vi "Calibrate Stereo Vision System (mod).vi"() -> ()   [LabVIEW 2014]
doc: "This example acquires images and demonstrates the binocular stereo vision algorithms installed with NI Vision Development Module. This example requires NI-IMAQdx. Refer to the Detailed Help for more information."
uses:
  SubVIs/Stereo - Calibration Manager Function.ctl
  <vilib>/vision/Stereo.llb/IMAQ Binocular Reference Coordinate System.ctl
  SubVIs/Stereo - Global Variables.vi
  <vilib>/vision/NI_Vision_Development_Module.lvlib
panel:
  in  "Process Band":bool
  out "Unit":string
  in  "Units":string[](array[string])=["", "Angström", "Micrometer", "Millimeter", "Centimeter", "Meter", "Kilometer", "Microinch", "Inch", "Feet", "Nautical miles", "Standard miles", "Steps"]
  out "Depth":dbl caption="Depth:"
  in  "Interpolate Disparity":bool=TRUE
  in  "Overlay Horizontal Lines":bool
  in  "View":enum16{"Acquired Images", "Rectified Images"}(ring)
  out "Grid Descriptor":cluster{"X Step":sgl, "Y Step":sgl, "Unit":T1}={"X Step"=1.0, "Y Step"=1.0, "Unit"=enum."Inch"}
  out "Grid Size":cluster{"X":i32, "Y":i32}
  in  "Live Image":bool=TRUE
  out "Calibration Status":u16(ring)
  in  "Display":enum16{"Disparity Image", "Depth Image"}(ring)
  in  "Relative Coordinate System":T2
  out "Image":sgl[][](graph) caption="Grid Coverage"
  in  "Exit":bool
  in  "Tab Control":T3(tab)
  out "Grid Coverage":T5
  in  "Save Single Calibrations":bool
  out "Quality":T6 caption="Stereo Calibration Quality" {"Rectification Quality 2" format="%#.5g"; "Rectification Quality" format="%#.5g"; "Calibration Quality" format="%#.5g"; "Max Distance" format="%#.4g"}
  in  "Save Grid Images":bool
  out "Scrollbar":u8(slide) caption="Acquire image in..." max=50 scale=0.0..100.0
  in  "Save Stereo Calibration":bool
  in  "Scaling Factor":sgl=1.0 min=0 max=1 step=0.1
  in  "Load":bool
  in  "Calibrate":bool
  out "Instruction Images":u16(ring) caption="Grid Orientation"
  out "Instructions":string
  in  "Time Lapse":u16=4 caption="Image Acquisition Time Lapse" min=1 max=60 step=1
  out "Grid Valid":bool=TRUE
  out "Calibration Grids":cluster{"Left Image":T4, "Right Image":T4}[](array[cluster]) caption="Left Calibration Grids"
  in  "Show":enum16{"Grid Coverage", "Calibration Grids"}(ring)
  in  "Max Depth (SGBM)":sgl=45.0 caption="Maximum Depth"
  in  "Correspondence Options SGBM":T7={"Method"=0, "Window Size"=15.0, "Minimum Disparity"=0.0, "Number of Disparity"=144.0, "P1"=100.0, "P2"=500.0, "Full DP"=FALSE, "Max Left Right Disparity"=5.0, "Subpixel"=TRUE, "Invalid Disparity Replace Value"=-16.0} caption="Correspondence Options" {"Method" items=["SAD"]; "Number of Disparity" min=16.0 step=16.0; "Window Size" min=5.0 max=255.0 step=2.0}
  in  "Postfilter Options SGBM":T8={"Texture Threshold"=0.0, "Uniqueness Ratio"=0.0, "Speckle Window Size"=5.0, "Speckle Range"=200.0} caption="Postfilter Options" {"Speckle Range" min=0.0; "Speckle Window Size" min=0.0; "Uniqueness Ratio" min=0.0 max=100.0; "Texture Threshold" min=0.0}
  in  "Filter Cap":u32=32
  in  "Correspondence Options BM":T9={"Method"=0, "Window Size"=25.0, "Minimum Disparity"=0.0, "Number of Disparity"=144.0, "Left - Right Check"=5.0, "Subpixel"=TRUE, "Invalid Disparity Replace Value"=-16.0} caption="Correspondence Options" {"Method" items=["SAD"]; "Number of Disparity" min=16.0 step=16.0; "Window Size" min=5.0 max=255.0 step=2.0}
  in  "Postfilter Options BM":T8={"Texture Threshold"=0.0, "Uniqueness Ratio"=0.0, "Speckle Window Size"=5.0, "Speckle Range"=200.0} caption="Postfilter Options" {"Speckle Range" min=0.0; "Speckle Window Size" min=0.0; "Uniqueness Ratio" min=0.0 max=100.0 step=1.0; "Texture Threshold" min=0.0}
  in  "Prefilter Options":T10={"Filter Type"=2, "Filter Size"=9.0, "Filter Cap"=31.0} {"Filter Type" items=["None", "Normal Response", "Sobel"]; "Filter Cap" min=1.0 max=63.0 step=1.0; "Filter Size" min=5.0 max=255.0 step=2.0}
  in  "Max Depth (BM)":sgl=45.0 caption="Maximum Depth"
  out "Right Image":T4(plugin-control)
  out "Left Image":T4(plugin-control)
  # "Overview: Demonstrate how to calibrate a stereo system and compute a depth image.\nRequirements: LabVIEW Full Development System, NI-IMAQdx and Vision Development Module\nNote: This example does not run on LabVIEW Real Time"
  # "s"
  # "Right Calibration Grids"
  # "Set the Maximum Depth corresponding to your setting:"
  # "Set the Maximum Depth corresponding to your setting:"
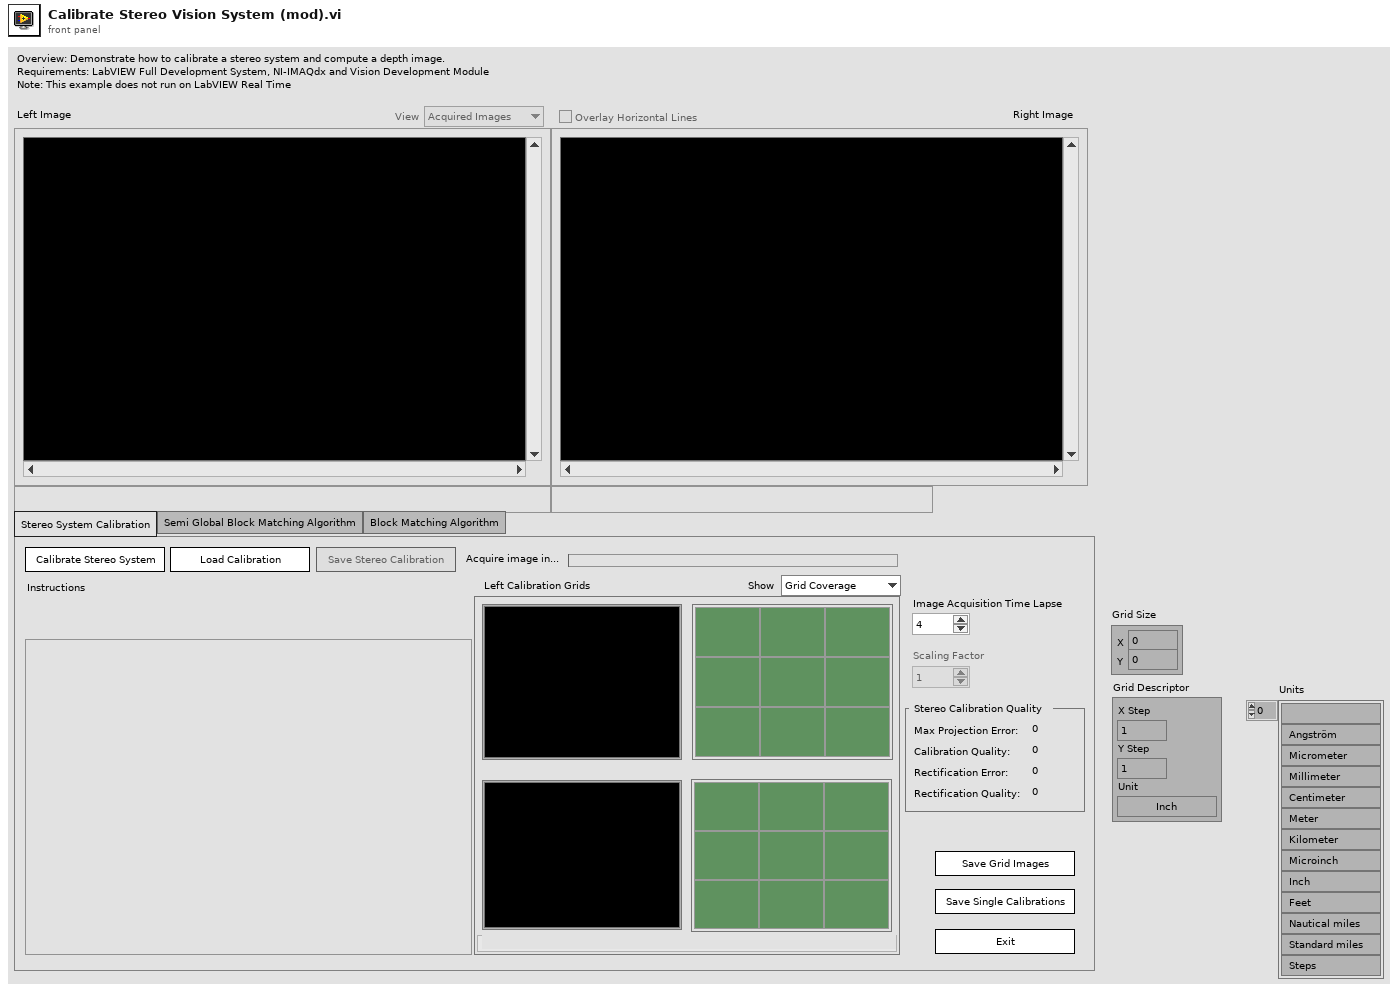
[diagram p1: front panel]
types:
  T1 = typedef "Image Unit" = enum32{"Undefined", "Angström", "Micrometer", "Millimeter", "Centimeter", "Meter", "Kilometer", "Microinch", "Inch", "Feet", "Nautical miles", "Standard miles", "Steps"}
  T2 = cluster{"Translation":cluster{"X":dbl, "Y":dbl, "Z":dbl}, "Rotation":cluster{"X":dbl, "Y":dbl, "Z":dbl}}
  T3 = enum32{"Stereo System Calibration", "Semi Global Block Matching Algorithm", "Block Matching Algorithm"}
  T4 = typedef "IMAQ Image.ctl" = refnum<image>
  T5 = cluster{"Left Image":T4, "Left Grid Coverage":bool[][], "Left Grid Coverage 3":string[][], "Right Image":T4, "Left Grid Coverage 2":bool[][], "Left Grid Coverage 4":string[][]}
  T6 = cluster{"Max Distance":dbl, "Calibration Quality":dbl, "Rectification Quality":dbl, "Rectification Quality 2":dbl}
  T7 = cluster{"Method":u16, "Window Size":dbl, "Minimum Disparity":dbl, "Number of Disparity":dbl, "P1":dbl, "P2":dbl, "Full DP":bool, "Max Left Right Disparity":dbl, "Subpixel":bool, "Invalid Disparity Replace Value":dbl}
  T8 = cluster{"Texture Threshold":dbl, "Uniqueness Ratio":dbl, "Speckle Window Size":dbl, "Speckle Range":dbl}
  T9 = cluster{"Method":u16, "Window Size":dbl, "Minimum Disparity":dbl, "Number of Disparity":dbl, "Left - Right Check":dbl, "Subpixel":bool, "Invalid Disparity Replace Value":dbl}
  T10 = cluster{"Filter Type":u16, "Filter Size":dbl, "Filter Cap":dbl}
  T11 = typedef "Stereo - Calibration Manager Function.ctl" = enum16{"Init", "Add Grid Images", "Get Images", "Dispose"}
  T12 = enum32{"Zero Order", "Bilinear", "Quadratic", "Cubic", "Bilinear Fixed"}
  T13 = typedef "IMAQ Binocular Reference Coordinate System.ctl" = enum32{" Left Camera", "Right Camera"}
  T14 = cluster{"Learn Lookup Table?":bool, "Render to original image?":bool, "Scaling Factor":sgl}
  T15 = enum8{"Enabled", "Disabled", "Disabled and Grayed Out"}
  T16 = enum32{"Page Enabled", "Page Disabled", "Page Disabled & Grayed"}
  T17 = typedef "Image Type" = u32
  T18 = typedef "IMAQ Binocular Stereo Session.ctl" = refnum<k1>
  T19 = typedef "Calibration Reference Points.ctl" = cluster{"Pixel Coordinates":cluster{"X":dbl, "Y":dbl}[], "Real World Coordinates":cluster{"X":dbl, "Y":dbl}[], "Unit":T1, "Image Size":cluster{"X":u32, "Y":u32}}
  T20 = cluster{"Image (dup)":T4, "Reference Points":T19}
  T21 = cluster{"Max. Projection Error":dbl, "Calibration Quality":dbl, "Max. Rectification Error":dbl, "Rectification Quality":dbl}
  T22 = typedef "LVPoint32TypeDef.ctl" = cluster{"Horizontal":i32, "Vertical":i32}
  T23 = cluster{"Max Depth (BM)":sgl, "Max Depth (BM)":sgl}
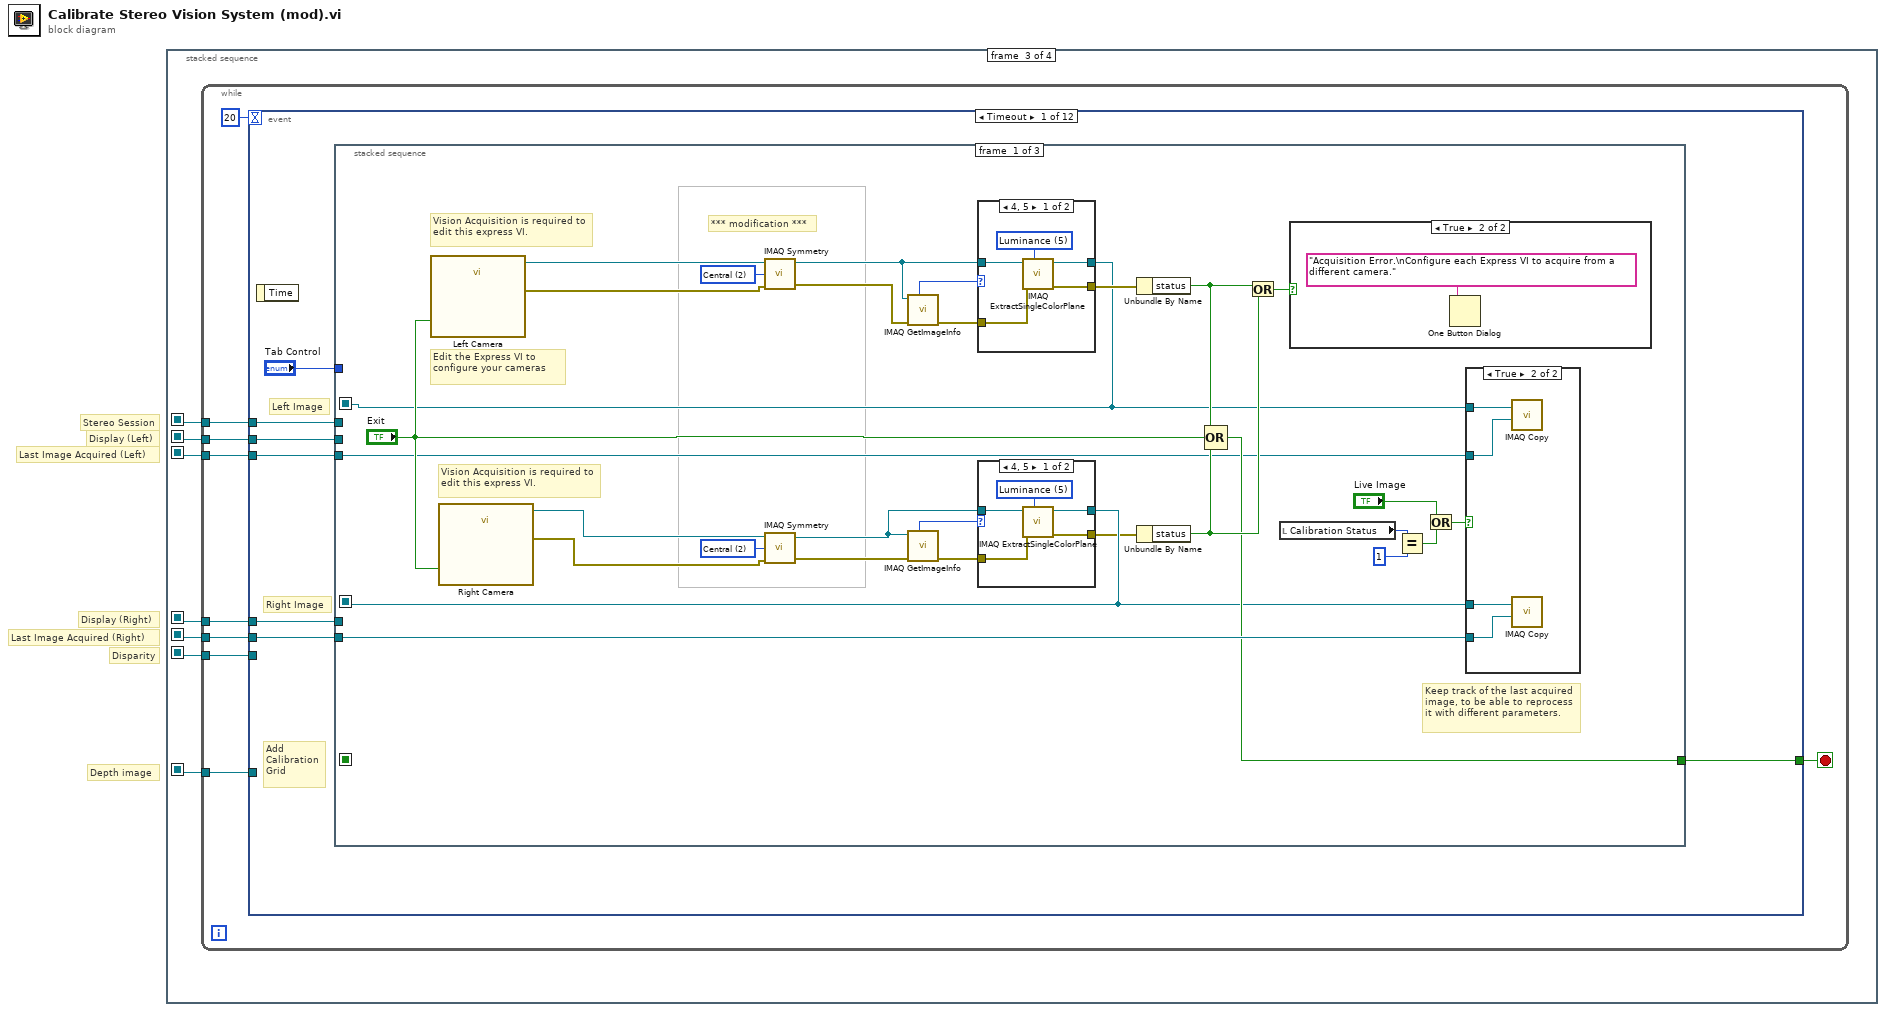
[diagram p0: block diagram]
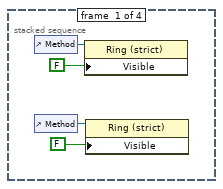
[diagram p2: hidden frame]
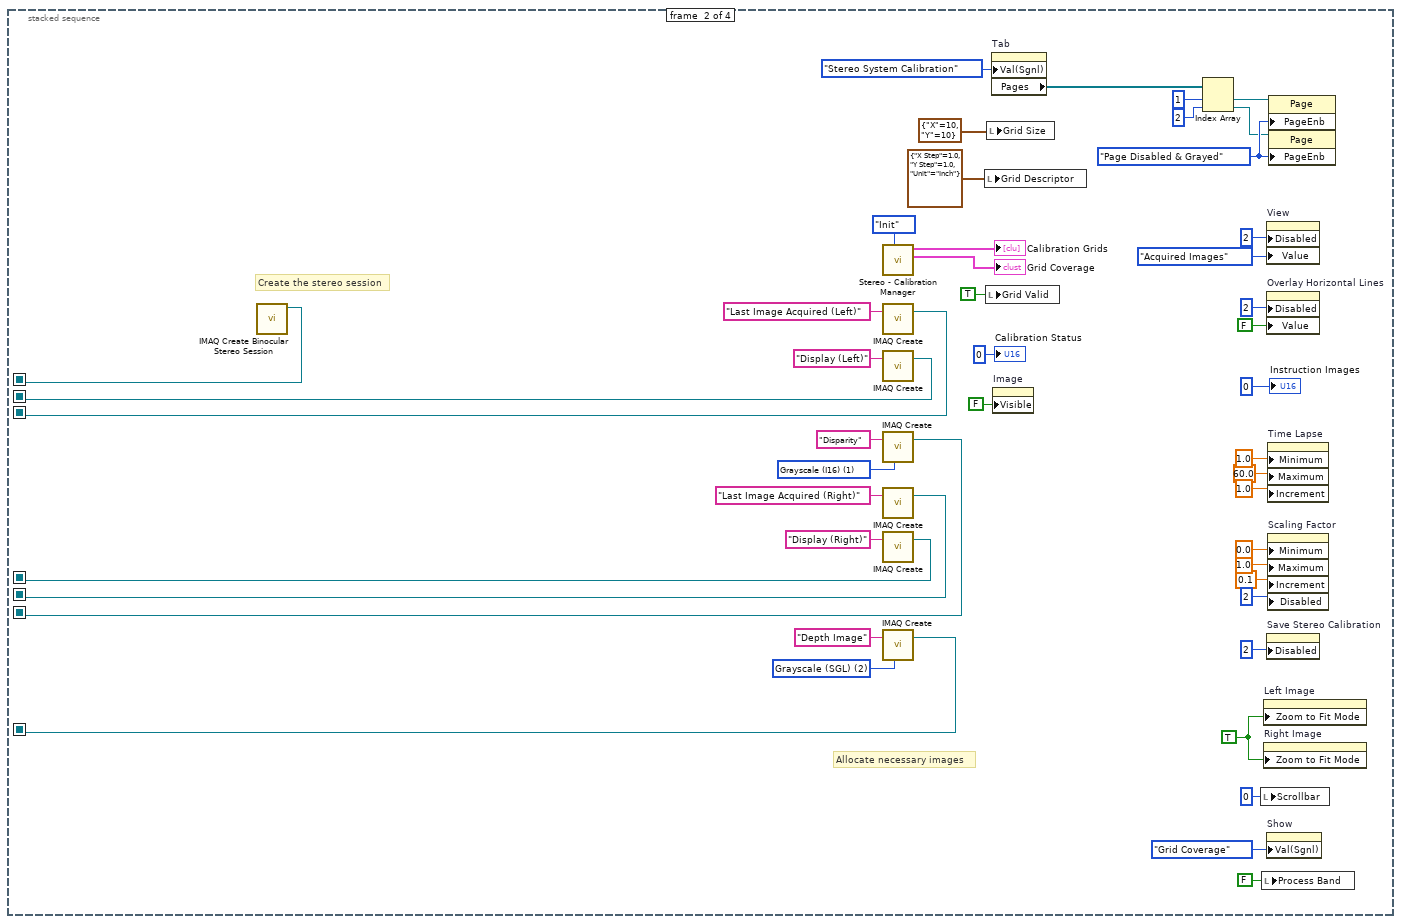
[diagram p3: hidden frame]
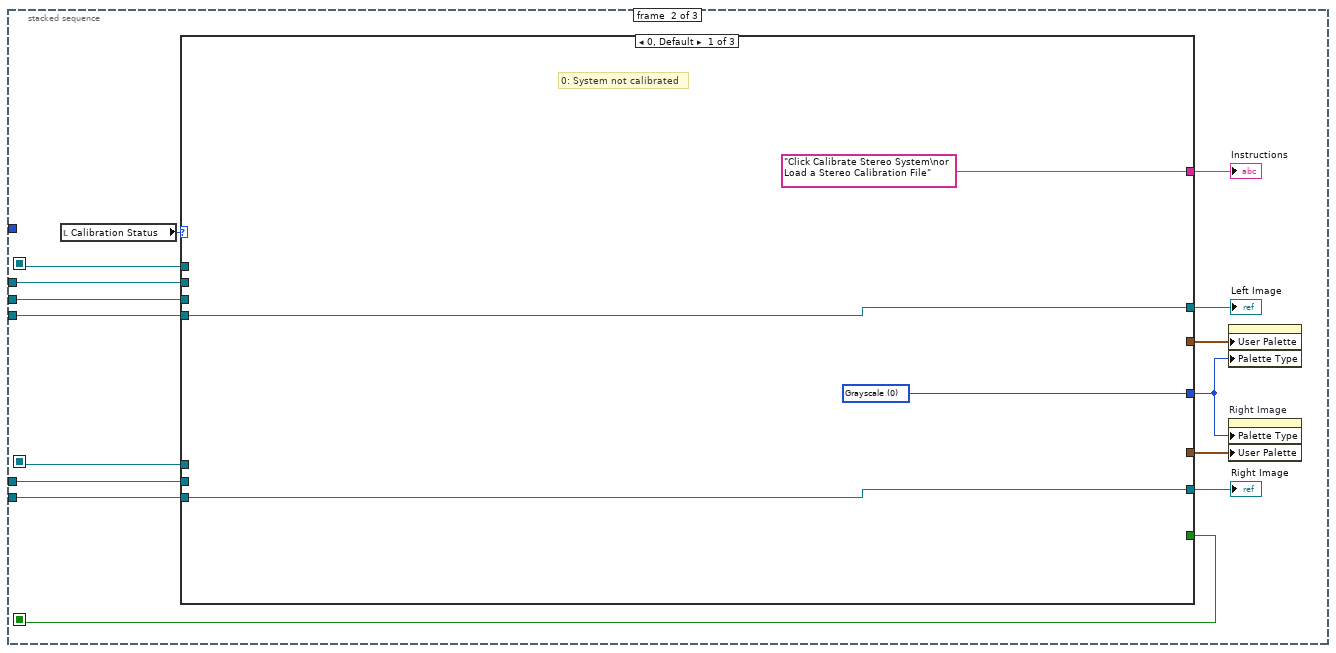
[diagram p8: hidden frame]
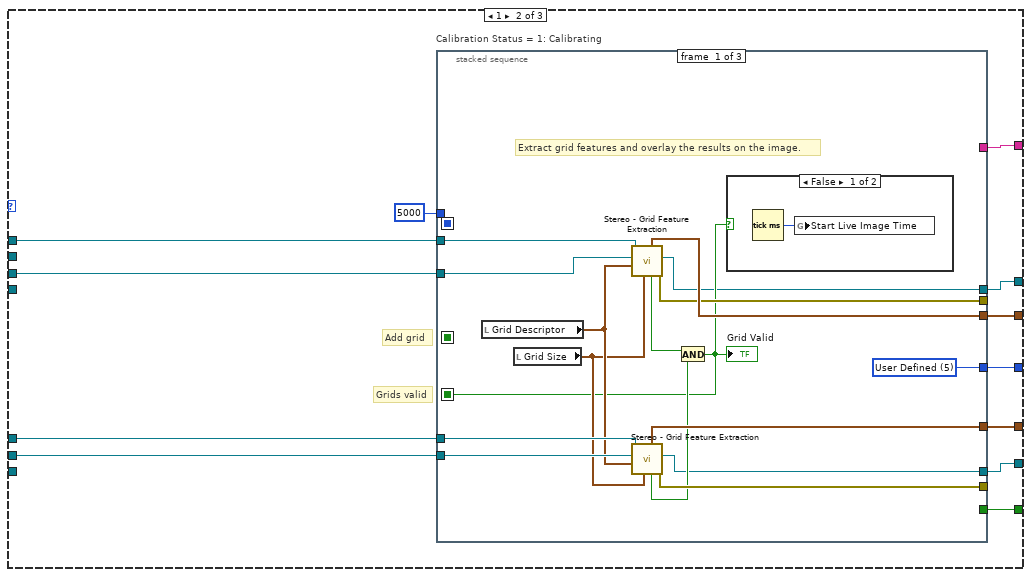
[diagram p9: hidden frame]
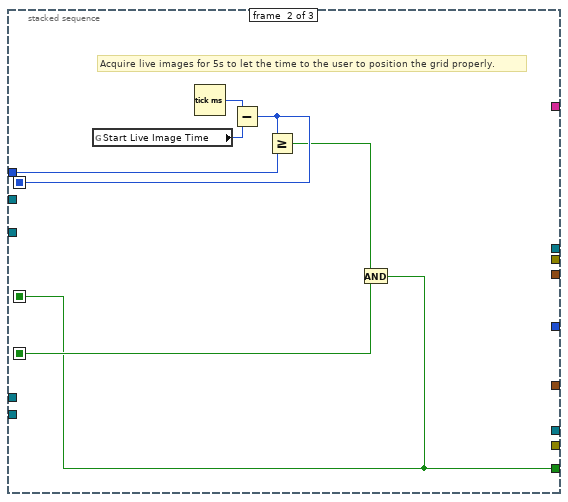
[diagram p11: hidden frame]
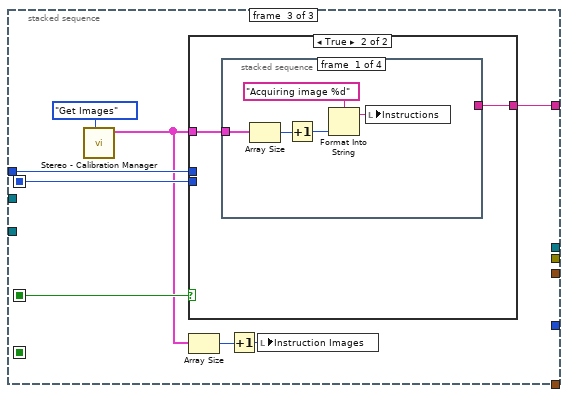
[diagram p12: hidden frame]
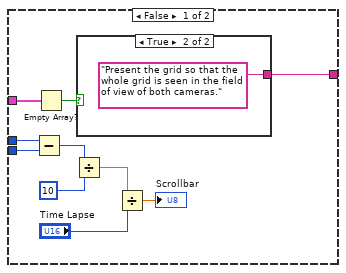
[diagram p13: hidden frame]
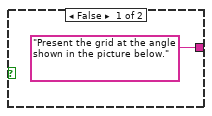
[diagram p14: hidden frame]
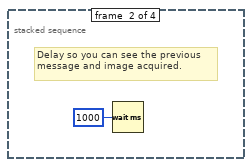
[diagram p15: hidden frame]
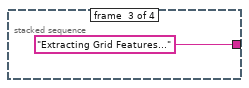
[diagram p16: hidden frame]
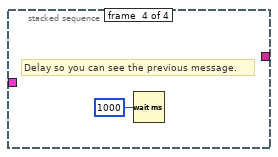
[diagram p17: hidden frame]
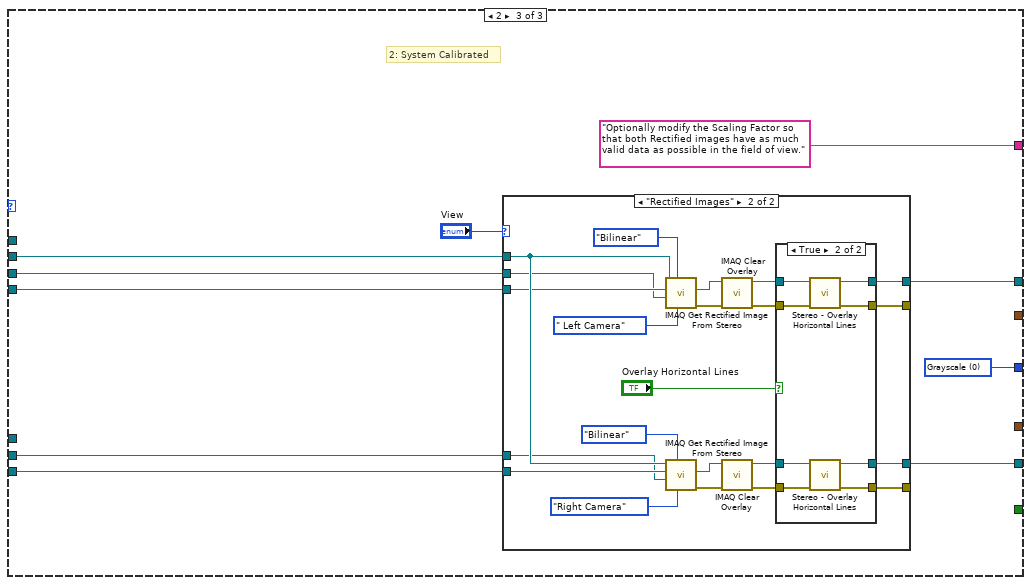
[diagram p18: hidden frame]
diagram:
  # "Depth image"
  # "Last Image Acquired (Right)"
  # "Disparity"
  # "Display (Right)"
  # "Display (Left)"
  # "Last Image Acquired (Left)"
  # "Stereo Session"
  n1 = stacked-sequence {
    seq-local: [_ w49 _ _] -> [_ _ w58 w612]
    seq-local: [_ w48 _ _] -> [_ _ w57 w610]
    seq-local: [_ w47 _ _] -> [_ _ w56 w613]
    seq-local: [_ w42 _ _] -> [_ _ w54 w609]
    seq-local: [_ w43 _ _] -> [_ _ w55 w611]
    seq-local: [_ w40 _ _] -> [_ _ w53 w608]
    seq-local: [_ w36 _ _] -> [_ _ w52 w606]
    frame #0 {
      n2 = control-ref of="Method"() -> (w4:refnum<vi>)
      n3 = control-ref of="Method"() -> (w1:refnum<vi>)
      n4 = property class="Ring (strict)"(reference=w4, "Visible"=FALSE) -> ()  [unwired: 1 in, 2 out]
      n5 = property class="Ring (strict)"(reference=w1, "Visible"=FALSE) -> ()  [unwired: 1 in, 2 out]
    }
    frame #1 {
      w12 = TRUE ("Zoom to Fit Mode")
      w30 = T16."Page Disabled & Grayed" ("Page Enabled State")
      w37 = T17 2 items=["Grayscale (U8)", "Grayscale (I16)", "Grayscale (SGL)", "Complex (CSG)", "RGB (U32)", "HSL (U32)", "RGB (U64)", "Grayscale (U16)"] ("Image Type")
      w39 = T17 1 items=["Grayscale (U8)", "Grayscale (I16)", "Grayscale (SGL)", "Complex (CSG)", "RGB (U32)", "HSL (U32)", "RGB (U64)", "Grayscale (U16)"] ("Image Type")
      # "Allocate necessary images"
      # "Create the stereo session"
      n6 = call "IMAQ Create Binocular Stereo Session"() -> ("Binocular Stereo Session Out"=w47:T18)  [unwired: 1 in, 10 out]
      n7 = call "Stereo - Calibration Manager.vi"("Function"=Stereo_-_Calibration_Manager_Function."Init") -> ("Grid Coverage"=→"Grid Coverage":T5, "Grid Images out"=→"Calibration Grids":cluster{"Left Image":T4, "Right Image":T4}[])  [unwired: 2 in, 7 out]
      n8 = call "IMAQ Create"("Image Name"="Last Image Acquired (Left)") -> ("New Image"=w43:T4)  [unwired: 3 in, 2 out]
      n9 = call "IMAQ Create"("Image Name"="Display (Left)") -> ("New Image"=w49:T4)  [unwired: 3 in, 2 out]
      n10 = call "IMAQ Create"("Image Name"="Disparity", "Image Type"=w39) -> ("New Image"=w40:T4)  [unwired: 2 in, 2 out]
      n11 = call "IMAQ Create"("Image Name"="Last Image Acquired (Right)") -> ("New Image"=w42:T4)  [unwired: 3 in, 2 out]
      n12 = call "IMAQ Create"("Image Name"="Display (Right)") -> ("New Image"=w48:T4)  [unwired: 3 in, 2 out]
      n13 = call "IMAQ Create"("Image Name"="Depth Image", "Image Type"=w37) -> ("New Image"=w36:T4)  [unwired: 2 in, 2 out]
      n14 = local write "Grid Descriptor"(cluster{"X Step":sgl, "Y Step":sgl, "Unit":T1} {"X Step"=1.0, "Y Step"=1.0, "Unit"=enum."Inch"} ("Grid Descriptor")) -> ()
      n15 = local write "Grid Valid"(TRUE ("Grid Valid")) -> ()
      n16 = local write "Grid Size"(cluster{"X":i32, "Y":i32} {"X"=10, "Y"=10} ("Grid Size")) -> ()
      n17 = property on="Tab" class="TabCtl (strict)"("Val(Sgnl)"=T3."Stereo System Calibration" ("Value (Signaling)")) -> ("Pages"=w34:refnum<vi>[])  [unwired: 2 in, 2 out]
      n18 = property on="Image" class="IntGraph (strict)"("Visible"=FALSE) -> ()  [unwired: 2 in, 2 out]
      n19 = Index Array(array=w34, index #1=1 ("index"), index #2=2 ("index")) -> (element #1=w33:refnum<vi>, element #2=w29:refnum<vi>)
      n20 = local write "Scrollbar"(u8 0 ("Scrollbar")) -> ()
      n21 = local write "Process Band"(FALSE ("Process Band")) -> ()
      n22 = property on="Left Image" class="ImageControl"("Zoom to Fit Mode"=w12) -> ()  [unwired: 2 in, 2 out]
      n23 = property on="Right Image" class="ImageControl"("Zoom to Fit Mode"=w12) -> ()  [unwired: 2 in, 2 out]
      n24 = property on="View" class="Enum (strict)"("Disabled"=u8 2, "Value"=enum16{"Acquired Images", "Rectified Images"}."Acquired Images" ("View")) -> ()  [unwired: 2 in, 2 out]
      n25 = property on="Overlay Horizontal Lines" class="Bool (strict)"("Disabled"=u8 2, "Value"=FALSE ("Overlay Horizontal Lines")) -> ()  [unwired: 2 in, 2 out]
      n26 = property on="Save Stereo Calibration" class="Bool"("Disabled"=u8 2) -> ()  [unwired: 2 in, 2 out]
      n27 = property on="Show" class="Enum (strict)"("Val(Sgnl)"=enum16{"Grid Coverage", "Calibration Grids"}."Grid Coverage" ("Value (Signaling)")) -> ()  [unwired: 2 in, 2 out]
      n28 = property on="Time Lapse" class="DigNum (strict)"("Minimum"=1.0 ("Data Entry Limits:Minimum"), "Maximum"=60.0 ("Data Entry Limits:Maximum"), "Increment"=1.0 ("Data Entry Limits:Increment")) -> ()  [unwired: 2 in, 2 out]
      n29 = property on="Scaling Factor" class="DigNum (strict)"("Minimum"=0.0 ("Data Entry Limits:Minimum"), "Maximum"=1.0 ("Data Entry Limits:Maximum"), "Increment"=0.1 ("Data Entry Limits:Increment"), "Disabled"=u8 2) -> ()  [unwired: 2 in, 2 out]
      n30 = property class="Page"(reference=w33, "PageEnb"=w30) -> ()  [unwired: 1 in, 2 out]
      n31 = property class="Page"(reference=w29, "PageEnb"=w30) -> ()  [unwired: 1 in, 2 out]
      "Calibration Status" <- u16 0 ("Status")
      "Instruction Images" <- u16 0 ("Grid Orientation")
    }
    frame #2 {
      n32 = while {
        tunnel: w58 -> [w66]
        tunnel: w57 -> [w65]
        tunnel: w56 -> [w63]
        tunnel: w55 -> [w62]
        tunnel: w54 -> [w61]
        tunnel: w53 -> [w60]
        tunnel: w52 -> [w59]
        stop <- w67 stop-if-true
        n33 = event shown="[0] Timeout" {
          selector: _ -> [_ _ _ _ _ _ _ _ _ _ _ _]
          dyn-events: _ -> [_ _ _ _ _ _ _ _ _ _ _ _]
          timeout: 20 -> [_ _ _ _ _ _ _ _ _ _ _ _]
          tunnel: [w74 _ _ _ _ _ _ _ _ _ _ _] -> w67
          tunnel: w66 -> [w73 _ _ _ _ _ _ _ _ _ _ _]
          tunnel: w65 -> [w72 _ _ _ _ _ _ _ _ _ _ _]
          tunnel: w63 -> [w69 _ _ w334 w383 w397 _ _ _ w461 _ w597]
          tunnel: w62 -> [w71 _ _ _ _ _ _ _ _ w460 _ _]
          tunnel: w61 -> [w70 _ _ _ _ _ _ _ _ w459 _ _]
          tunnel: w60 -> [_ _ _ _ _ _ _ _ _ w458 _ w596]
          tunnel: w59 -> [_ _ _ _ _ _ _ _ _ w451 _ _]
          event Timeout {
            # "Add\nCalibration\nGrid"
            # "Right Image"
            # "Left Image"
            n34 = event-data() -> ()  [unwired: 2 out]
            n35 = stacked-sequence {
              seq-local: [w75 _ _] -> [_ w135 w260]
              seq-local: [w90 _ _] -> [_ w133 w259]
              seq-local: [_ w137 _] -> [_ _ w256]
              tunnel: [w95 _ _] -> w74
              tunnel: w73 -> [_ w134 w258]
              tunnel: w72 -> [_ w132 w257]
              tunnel: w71 -> [w78 w126 _]
              tunnel: w70 -> [w104 w125 _]
              tunnel: w69 -> [_ w124 _]
              tunnel: "Tab Control" -> [_ _ w255]
              frame #0 {
                w76 = u32 2 items=["Horizontal", "Vertical", "Central", "1st Diagonal", "2nd Diagonal"] ("Type of Symmetry")
                w77 = u32 2 items=["Horizontal", "Vertical", "Central", "1st Diagonal", "2nd Diagonal"] ("Type of Symmetry")
                # "*** modification ***"
                # "Vision Acquisition is required to edit this express VI."
                # "Vision Acquisition is required to edit this express VI."
                # "Edit the Express VI to configure your cameras"
                # "Keep track of the last acquired image, to be able to reprocess it with different parameters."
                n36 = call "Left Camera"("Stop (F)"="Exit") -> ("Image Out"=w87:T4, "error out"=w84:errorcluster)  [unwired: 1 in, 24 out]
                n37 = call "Right Camera"("Stop (F)"="Exit") -> ("Image Out"=w81:T4, "error out"=w80:errorcluster)  [unwired: 1 in, 24 out]
                n38 = call "IMAQ Symmetry"("error in (no error)"=w84, "Type of Symmetry"=w76, "Image Src"=w87) -> ("error out"=w85:errorcluster, "Image Dst Out"=w86:T4)  [unwired: 2 in]
                n39 = call "IMAQ Symmetry"("error in (no error)"=w80, "Type of Symmetry"=w77, "Image Src"=w81) -> ("error out"=w82:errorcluster, "Image Dst Out"=w83:T4)  [unwired: 2 in]
                n40 = call "IMAQ GetImageInfo"("error in (no error)"=w85, "Image"=w86) -> ("error out"=w93:errorcluster, "Image Type"=w94:T17)  [unwired: 8 out]
                n41 = call "IMAQ GetImageInfo"("error in (no error)"=w82, "Image"=w83) -> ("error out"=w91:errorcluster, "Image Type"=w88:T17)  [unwired: 8 out]
                n42 = case shown="4, 5" w94 {
                  tunnel: w86 -> [w116 w118]
                  tunnel: [w114 w118] -> w75
                  tunnel: w93 -> [w113 w117]
                  tunnel: [w112 w117] -> w92
                  frame 4, 5 {
                    w115 = 5 items=["Red", "Green", "Blue", "Hue", "Saturation", "Luminance", "Value", "Intensity"] ("Color Plane")
                    n43 = call "IMAQ ExtractSingleColorPlane"("Color Plane"=w115, "error in (no error)"=w113, "Image Src"=w116) -> ("error out"=w112:errorcluster, "Image Dst Out"=w114:T4)  [unwired: 1 in, 6 out]
                  }
                  frame Default {
                  }
                }
                n44 = case shown="4, 5" w88 {
                  tunnel: w83 -> [w109 w111]
                  tunnel: [w107 w111] -> w90
                  tunnel: w91 -> [w106 w110]
                  tunnel: [w105 w110] -> w89
                  frame 4, 5 {
                    w108 = 5 items=["Red", "Green", "Blue", "Hue", "Saturation", "Luminance", "Value", "Intensity"] ("Color Plane")
                    n45 = call "IMAQ ExtractSingleColorPlane"("Color Plane"=w108, "error in (no error)"=w106, "Image Src"=w109) -> ("error out"=w105:errorcluster, "Image Dst Out"=w107:T4)  [unwired: 1 in, 6 out]
                  }
                  frame Default {
                  }
                }
                n46 = Unbundle By Name(w92) -> ("status"=w97:bool)
                n47 = Unbundle By Name(w89) -> ("status"=w96:bool)
                n48 = Compound Arithmetic op=OR(w97, "Exit", w96) -> (w95:bool)
                n49 = Or(x=w97, y=w96) -> (x .or. y?=w98:bool)
                n50 = local read "Calibration Status"() -> (w103:u16)
                n51 = case shown="True" w98 {
                  frame False {
                  }
                  frame True {
                    n52 = One Button Dialog(message="Acquisition Error.\nConfigure each Express VI to acquire from a different camera.") -> ()  [unwired: 2 out]
                  }
                }
                n53 = Equal?(x=w103, y=u16 1) -> (x = y?=w100:bool)
                n54 = Or(x="Live Image", y=w100) -> (x .or. y?=w99:bool)
                n55 = case shown="True" w99 {
                  tunnel: w75 -> [_ w123]
                  tunnel: w78 -> [_ w122]
                  tunnel: w90 -> [_ w121]
                  tunnel: w104 -> [_ w120]
                  frame False {
                  }
                  frame True {
                    n56 = call "IMAQ Copy"("Image Dst"=w122, "Image Src"=w123) -> ()  [unwired: 1 in, 5 out]
                    n57 = call "IMAQ Copy"("Image Dst"=w120, "Image Src"=w121) -> ()  [unwired: 1 in, 5 out]
                  }
                }
              }
              frame #1 {
                n58 = local read "Calibration Status"() -> (w136:u16)
                n59 = case shown="0, Default" w136 {
                  tunnel: ["Click Calibrate Stereo System\nor Load a Stereo Calibration File" ("Instructions") w154 "Optionally modify the Scaling Factor so that both Rectified images have as much valid data as possible in the field of view." ("Instructions")] -> w138
                  tunnel: [_ w153 _] -> w137
                  tunnel: w135 -> [_ w152 _]
                  tunnel: w134 -> [_ w151 w211]
                  tunnel: w133 -> [_ w150 _]
                  tunnel: w132 -> [_ w149 w210]
                  tunnel: [w141 w148 w215] -> w128
                  tunnel: [w140 w147 w213] -> w129
                  tunnel: [_ w146 _] -> w131
                  tunnel: [_ w145 _] -> w130
                  tunnel: [w142 w144 w218] -> w127
                  tunnel: w126 -> [w141 _ w216]
                  tunnel: w125 -> [w140 _ w214]
                  tunnel: w124 -> [_ _ w212]
                  frame 0, Default {
                    w142 = u32 0 items=["Grayscale", "Binary", "Gradient", "Rainbow", "Temperature", "User Defined"] ("Palette:Palette Type")
                    # "0: System not calibrated"
                  }
                  frame 1 {
                    # "Add grid"
                    # "Grids valid"
                    n60 = stacked-sequence "Calibration Status = 1: Calibrating" {
                      seq-local: [w157 _ _] -> [_ w173 _]
                      seq-local: [_ w172 _] -> [_ _ w186]
                      seq-local: [_ w175 _] -> [_ _ w184]
                      tunnel: [_ _ w183] -> w154
                      tunnel: [_ w172 _] -> w153
                      tunnel: w152 -> [w170 _ _]
                      tunnel: w151 -> [w169 _ _]
                      tunnel: w150 -> [w168 _ _]
                      tunnel: w149 -> [w167 _ _]
                      tunnel: [w156 _ _] -> w148
                      tunnel: [w155 _ _] -> w147
                      tunnel: [w166 _ _] -> w146
                      tunnel: [w165 _ _] -> w145
                      tunnel: [w164 _ _] -> w144
                      tunnel: [w163 _ _] -> _
                      tunnel: [w162 _ _] -> _
                      tunnel: u32 5000 ("y") -> [_ w176 w185]
                      frame #0 {
                        w164 = u32 5 items=["Grayscale", "Binary", "Gradient", "Rainbow", "Temperature", "User Defined"] ("Palette:Palette Type")
                        # "Extract grid features and overlay the results on the image."
                        n61 = local read "Grid Descriptor"() -> (w161:cluster{"X Step":sgl, "Y Step":sgl, "Unit":T1})
                        n62 = local read "Grid Size"() -> (w160:cluster{"X":i32, "Y":i32})
                        n63 = call "Stereo - Grid Feature Extraction.vi"("Grid Size"=w160, "Grid Descriptor"=w161, "Display Image in"=w169, "Image in"=w170) -> ("error out"=w163:errorcluster, "Display Image out"=w156:T4, "Valid Grid"=w159:bool, "Color Palette"=w165:cluster{"Red":u8, "Green":u8, "Blue":u8}[])  [unwired: 2 in, 2 out]
                        n64 = call "Stereo - Grid Feature Extraction.vi"("Grid Size"=w160, "Grid Descriptor"=w161, "Display Image in"=w167, "Image in"=w168) -> ("error out"=w162:errorcluster, "Display Image out"=w155:T4, "Valid Grid"=w158:bool, "Color Palette"=w166:cluster{"Red":u8, "Green":u8, "Blue":u8}[])  [unwired: 2 in, 2 out]
                        n65 = And(x=w159, y=w158) -> (x .and. y?=w157:bool)
                        "Grid Valid" <- w157
                        n66 = case shown="False" w157 {
                          frame False {
                            n67 = Tick Count (ms)() -> (millisecond timer value=w171:u32)
                            n68 = global write "Stereo - Global Variables.vi" "Start Live Image Time"(w171) -> ()
                          }
                          frame True {
                          }
                        }
                      }
                      frame #1 {
                        # "Acquire live images for 5s to let the time to the user to position the grid properly."
                        n69 = global read "Stereo - Global Variables.vi" "Start Live Image Time"() -> (w177:u32)
                        n70 = Tick Count (ms)() -> (millisecond timer value=w178:u32)
                        n71 = Subtract(x=w178, y=w177) -> (x-y=w175:u32)
                        n72 = Greater Or Equal?(x=w175, y=w176) -> (x >= y?=w174:bool)
                        n73 = And(x=w174, y=w173) -> (x .and. y?=w172:bool)
                      }
                      frame #2 {
                        n74 = call "Stereo - Calibration Manager.vi"("Function"=Stereo_-_Calibration_Manager_Function."Get Images") -> ("Grid Images out"=w179:cluster{"Left Image":T4, "Right Image":T4}[])  [unwired: 2 in, 8 out]
                        n75 = case shown="True" w186 {
                          tunnel: w184 -> [w195 _]
                          tunnel: w185 -> [w196 _]
                          tunnel: [w187 w200] -> w183
                          tunnel: w179 -> [w192 w199]
                          frame False {
                            n76 = Subtract(x=w196, y=w195) -> (x-y=w194:u32)
                            n77 = Empty Array?(array=w192) -> (empty?=w191:bool)
                            n78 = Divide(x=w194, y=u32 10) -> (x/y=w189:dbl)
                            n79 = case shown="True" w191 {
                              tunnel: ["Present the grid at the angle shown in the picture below." ("Instructions") "Present the grid so that the whole grid is seen in the field of view of both cameras." ("Instructions")] -> w187
                              frame False {
                              }
                              frame True {
                              }
                            }
                            n80 = Divide(x=w189, y="Time Lapse") -> (x/y=→"Scrollbar":dbl)
                          }
                          frame True {
                            n81 = stacked-sequence {
                              tunnel: [_ _ "Extracting Grid Features..." ("Instructions") _] -> w200
                              tunnel: w199 -> [w201 _ _ _]
                              frame #0 {
                                n82 = Array Size(array=w201) -> (size(s)=w205:i32)
                                n83 = Increment(x=w205) -> (x+1=w203:i32)
                                n84 = Format Into String(format string="Acquiring image %d" ("Instructions"), w203) -> (resulting string=w202:string)  [unwired: 2 in, 1 out]
                                n85 = local write "Instructions"(w202) -> ()
                              }
                              frame #1 {
                                # "Delay so you can see the previous message and image acquired."
                                n86 = Wait (ms)(milliseconds to wait=u32 1000) -> ()  [unwired: 1 out]
                              }
                              frame #2 {
                              }
                              frame #3 {
                                # "Delay so you can see the previous message."
                                n87 = Wait (ms)(milliseconds to wait=u32 1000) -> ()  [unwired: 1 out]
                              }
                            }
                          }
                        }
                        n88 = Array Size(array=w179) -> (size(s)=w181:i32)
                        n89 = Increment(x=w181) -> (x+1=w180:i32)
                        n90 = local write "Instruction Images"(w180) -> ()
                      }
                    }
                  }
                  frame 2 {
                    w218 = u32 0 items=["Grayscale", "Binary", "Gradient", "Rainbow", "Temperature", "User Defined"] ("Palette:Palette Type")
                    # "2: System Calibrated"
                    n91 = case shown="\"Rectified Images\"" "View" {
                      tunnel: w216 -> [w219 w239]
                      tunnel: [w219 w234] -> w215
                      tunnel: w214 -> [w220 w238]
                      tunnel: [w220 w233] -> w213
                      tunnel: w212 -> [_ w242]
                      tunnel: w211 -> [_ w237]
                      tunnel: w210 -> [_ w236]
                      tunnel: [_ w235] -> _
                      tunnel: [_ w232] -> _
                      frame "Acquired Images", Default {
                      }
                      frame "Rectified Images" {
                        n92 = call "IMAQ Get Rectified Image From Stereo"("Reference Coordinate System"=IMAQ_Binocular_Reference_Coordinate_System." Left Camera", "Interpolation Type"=T12."Bilinear", "Image Dst"=w237, "Image Src"=w239, "Binocular Stereo Session"=w242) -> ("error out"=w230:errorcluster, "Image Dst Out"=w228:T4)  [unwired: 1 in, 4 out]
                        n93 = call "IMAQ Get Rectified Image From Stereo"("Reference Coordinate System"=IMAQ_Binocular_Reference_Coordinate_System."Right Camera", "Interpolation Type"=T12."Bilinear", "Image Dst"=w236, "Image Src"=w238, "Binocular Stereo Session"=w242) -> ("error out"=w224:errorcluster, "Image Dst Out"=w226:T4)  [unwired: 1 in, 4 out]
                        n94 = call "IMAQ Clear Overlay"("error in (no error)"=w230, "Image"=w228) -> ("error out"=w229:errorcluster, "Image Out"=w227:T4)  [unwired: 1 in, 7 out]
                        n95 = call "IMAQ Clear Overlay"("error in (no error)"=w224, "Image"=w226) -> ("error out"=w223:errorcluster, "Image Out"=w225:T4)  [unwired: 1 in, 7 out]
                        n96 = case shown="True" "Overlay Horizontal Lines" {
                          tunnel: w229 -> [w245 w254]
                          tunnel: [w245 w253] -> w235
                          tunnel: w227 -> [w246 w252]
                          tunnel: [w246 w251] -> w234
                          tunnel: w225 -> [w244 w250]
                          tunnel: [w244 w249] -> w233
                          tunnel: w223 -> [w243 w248]
                          tunnel: [w243 w247] -> w232
                          frame False {
                          }
                          frame True {
                            n97 = call "Stereo - Overlay Horizontal Lines.vi"("error in (no error)"=w254, "Rectified Image in"=w252) -> ("error out"=w253:errorcluster, "Rectified Image out"=w251:T4)  [unwired: 1 in, 7 out]
                            n98 = call "Stereo - Overlay Horizontal Lines.vi"("error in (no error)"=w248, "Rectified Image in"=w250) -> ("error out"=w247:errorcluster, "Rectified Image out"=w249:T4)  [unwired: 1 in, 7 out]
                          }
                        }
                      }
                    }
                  }
                }
                "Instructions" <- w138
                "Left Image" <- w128
                "Right Image" <- w129
                n99 = property on="Left Image" class="ImageControl"("User Palette"=w130, "Palette Type"=w127) -> ()  [unwired: 2 in, 2 out]
                n100 = property on="Right Image" class="ImageControl"("Palette Type"=w127, "User Palette"=w131) -> ()  [unwired: 2 in, 2 out]
              }
              frame #2 {
                n101 = case shown="\"Stereo System Calibration\"" w255 {
                  tunnel: w260 -> [w265 _]
                  tunnel: w259 -> [w264 _]
                  tunnel: w258 -> [w263 _]
                  tunnel: w257 -> [w262 _]
                  tunnel: w256 -> [w261 _]
                  frame "Stereo System Calibration" {
                    n102 = case shown="True" w261 {
                      tunnel: w265 -> [_ w269]
                      tunnel: w264 -> [_ w268]
                      tunnel: w263 -> [_ w267]
                      tunnel: w262 -> [_ w266]
                      frame False {
                      }
                      frame True {
                        n103 = stacked-sequence {
                          tunnel: w269 -> [w286 _]
                          tunnel: w268 -> [w285 _]
                          tunnel: w267 -> [w284 _]
                          tunnel: w266 -> [w283 _]
                          frame #0 {
                            # "Extract the features from the grids."
                            n104 = local read "Grid Descriptor"() -> (w270:cluster{"X Step":sgl, "Y Step":sgl, "Unit":T1})
                            n105 = local read "Grid Size"() -> (w271:cluster{"X":i32, "Y":i32})
                            n106 = call "Stereo - Grid Feature Extraction.vi"("Grid Size"=w271, "Grid Descriptor"=w270, "Display Image in"=w284, "Image in"=w286) -> ("error out"=w273:errorcluster, "Reference Points"=w281:T19, "Image (dup)"=w282:T4, "Valid Grid"=w275:bool, "Color Palette"=w277:cluster{"Red":u8, "Green":u8, "Blue":u8}[])  [unwired: 2 in, 1 out]
                            n107 = call "Stereo - Grid Feature Extraction.vi"("Grid Size"=w271, "Grid Descriptor"=w270, "Display Image in"=w283, "Image in"=w285) -> ("error out"=w272:errorcluster, "Reference Points"=w279:T19, "Image (dup)"=w280:T4, "Valid Grid"=w274:bool, "Color Palette"=w276:cluster{"Red":u8, "Green":u8, "Blue":u8}[])  [unwired: 2 in, 1 out]
                            n108 = And(x=w275, y=w274) -> (x .and. y?=w278:bool)
                            n109 = case shown="True" w278 {
                              tunnel: w282 -> [_ w294]
                              tunnel: w281 -> [_ w293]
                              tunnel: w280 -> [_ w292]
                              tunnel: w279 -> [_ w291]
                              tunnel: w277 -> [_ w290]
                              tunnel: w276 -> [_ w289]
                              tunnel: w273 -> [_ _]
                              tunnel: w272 -> [_ _]
                              frame False {
                                n110 = flat-sequence {
                                frame #0 {
                                n111 = local write "Instructions"("Not Enough Dots Detected." ("Instructions")) -> ()
                                }
                                frame #1 {
                                # "Delay so you can see the message."
                                n112 = Wait (ms)(milliseconds to wait=u32 1000) -> ()  [unwired: 1 out]
                                }
                                }
                              }
                              frame True {
                                n113 = stacked-sequence {
                                seq-local: [_ _ w303 _] -> [_ _ _ w313]
                                tunnel: w294 -> [_ _ w311 _]
                                tunnel: w293 -> [_ _ w310 _]
                                tunnel: w292 -> [_ _ w308 _]
                                tunnel: w291 -> [_ _ w307 _]
                                tunnel: w290 -> [_ _ _ _]
                                tunnel: w289 -> [_ _ _ _]
                                frame #0 {
                                n114 = local write "Instructions"("Calibrating each camera..." ("Instructions")) -> ()
                                }
                                frame #1 {
                                # "Delay so you can see the instruction we just set in the previous frame."
                                n115 = Wait (ms)(milliseconds to wait=u32 500) -> ()  [unwired: 1 out]
                                }
                                frame #2 {
                                # "The grids are valid. Add them to the calibration manager and compute the camera models of each camera."
                                n116 = Bundle("Image (dup)"=w311, "Reference Points"=w310) -> (w309:T20)  [unwired: 1 out]
                                n117 = Bundle("Image (dup)"=w308, "Reference Points"=w307) -> (w306:T20)  [unwired: 1 out]
                                n118 = call "Stereo - Calibration Manager.vi"("Function"=Stereo_-_Calibration_Manager_Function."Add Grid Images", "Right Grid Image"=w306, "Left Grid Image"=w309) -> ("Calibration OK"=w303:bool, "Grid Coverage"=w297:T5, "Grid Images out"=w302:cluster{"Left Image":T4, "Right Image":T4}[])  [unwired: 6 out]
                                n119 = Array Size(array=w302) -> (size(s)=w301:i32)
                                n120 = local write "Grid Coverage"(w297) -> ()
                                n121 = Subtract(x=w301, y=2) -> (x-y=w299:i32)
                                n122 = Max & Min(x=w299, y=0) -> (max(x,y)=w305:i32)  [unwired: 1 out]
                                n123 = Build Array(w305) -> (w304:i32[])
                                n124 = property on="Calibration Grids" class="Arr (strict)"("Val(Sgnl)"=w302, "Index Values"=w304) -> ()  [unwired: 2 in, 2 out]
                                }
                                frame #3 {
                                n125 = case "If the single camera calibrations are OK,\nfire a Scaling Factor event to compute\nthe stereo calibration" shown="True" w313 {
                                frame False {
                                }
                                frame True {
                                n126 = property on="Scaling Factor" class="DigNum (strict)"("Val(Sgnl)"="Scaling Factor") -> ()  [unwired: 2 in, 2 out]
                                }
                                }
                                }
                                }
                              }
                            }
                          }
                          frame #1 {
                            # "Reset the Start Live Image tick count to start acquiring live images again."
                            n127 = Tick Count (ms)() -> (millisecond timer value=w315:u32)
                            n128 = global write "Stereo - Global Variables.vi" "Start Live Image Time"(w315) -> ()
                          }
                        }
                      }
                    }
                  }
                  frame Default {
                    n129 = local read "Live Image"() -> (w316:bool)
                    n130 = case shown="True" w316 {
                      frame False {
                      }
                      frame True {
                        # "If we're acquiring a live image, fire this event to process it."
                        n131 = property on="Prefilter Options" class="Clust (strict)"() -> ("Value"=w317:T10)  [unwired: 2 in, 2 out]
                        n132 = property on="Prefilter Options" class="Clust (strict)"("Val(Sgnl)"=w317) -> ()  [unwired: 2 in, 2 out]
                      }
                    }
                  }
                }
              }
            }
          }
          event "Calibrate": Value Change {
            n133 = event-data() -> ()  [unwired: 2 out]
            n134 = call "Stereo - Grid Parameters Dialog.vi"() -> ("Cancel Indicator"=w318:bool, "Grid Size out"=w319:cluster{"X":i32, "Y":i32}, "Grid Descriptor out"=w320:cluster{"X Step":sgl, "Y Step":sgl, "Unit":T1})  [unwired: 9 out]
            n135 = case shown="False" w318 {
              tunnel: w320 -> [w324 _]
              tunnel: w319 -> [w325 _]
              frame False {
                w329 = u16 1  # Calibrating...
                # "Initialize calibration manager."
                n136 = Unbundle By Name(w324) -> ("Unit"=w323:T1)
                n137 = call "Stereo - Calibration Manager.vi"("Function"=Stereo_-_Calibration_Manager_Function."Init") -> ("Grid Images out"=w326:cluster{"Left Image":T4, "Right Image":T4}[])  [unwired: 2 in, 8 out]
                n138 = Tick Count (ms)() -> (millisecond timer value=w328:u32)
                n139 = Index Array(array="Units", index=w323) -> (element=→"Unit":string)
                n140 = local write "Calibration Grids"(w326) -> ()
                n141 = global write "Stereo - Global Variables.vi" "Start Calibration Time"(w328) -> ()
                n142 = global write "Stereo - Global Variables.vi" "Start Live Image Time"(w328) -> ()
                n143 = property on="Calibration Status" class="Ring (strict)"("Value"=w329, "Blinking"=TRUE) -> ()  [unwired: 2 in, 2 out]
                "Grid Size" <- w325
                "Grid Descriptor" <- w324
              }
              frame True {
              }
            }
          }
          event "Show": Value Change {
            n144 = event-data() -> ("NewVal"=w332:enum16{"Grid Coverage", "Calibration Grids"})  [unwired: 1 out]
            n145 = Equal To 0?(x=w332) -> (x = 0?=w331:bool)
            n146 = property on="Grid Coverage" class="Clust (strict)"("Visible"=w331) -> ()  [unwired: 2 in, 2 out]
          }
          event "Scaling Factor": Value Change {
            n147 = event-data() -> ("NewVal"=w333:sgl)  [unwired: 1 out]
            n148 = stacked-sequence {
              seq-local: [_ _ w346 _] -> [_ _ _ w370]
              tunnel: w334 -> [_ _ w351 _]
              tunnel: w333 -> [_ _ w347 _]
              frame #0 {
                n149 = local write "Instructions"("Computing Stereo Calibration" ("Instructions")) -> ()
              }
              frame #1 {
                # "Delay so you can see the previous message."
                n150 = Wait (ms)(milliseconds to wait=u32 1000) -> ()  [unwired: 1 out]
              }
              frame #2 {
                # "Compute the stereo vision calibration"
                n151 = call "Stereo - Calibration Manager.vi"("Function"=Stereo_-_Calibration_Manager_Function."Get Images") -> ("Calibrated Images"=w349:T4[])  [unwired: 2 in, 8 out]
                n152 = Bundle By Name(cluster=T14 {"Learn Lookup Table?"=TRUE, "Render to original image?"=FALSE, "Scaling Factor"=0.0} ("Rectification Settings"), "Scaling Factor"=w347) -> (w339:T14)
                n153 = Index Array(array=w349) -> (element #1=w338:T4, element #2=w344:T4)  [unwired: 2 in]
                n154 = call "IMAQ GetImageSize"("Image"=w338) -> ("X Resolution"=w337:i32)  [unwired: 1 in, 4 out]
                n155 = call "Stereo - Corresponding Points Dialog.vi"("Right Image in"=w344, "Left Image in"=w338) -> ("Right Image out"=w343:T4, "Left Image out"=w345:T4)  [unwired: 8 out]
                n156 = call "IMAQ Learn Binocular Stereo Calibration"("Rectification Settings"=w339, "Right Calibration Template"=w343, "Left Calibration Template"=w345, "Binocular Stereo Session"=w351) -> ("error out"=w348:errorcluster, "Quality"=w342:T21, "Binocular Stereo Session (dup)"=w341:T18)  [unwired: 1 in, 4 out]
                "Quality" <- w342
                n157 = case shown="No Error" w348 {
                  selector: w348 -> [_ w368]
                  tunnel: [w355 w367] -> w346
                  tunnel: w342 -> [w356 _]
                  tunnel: w341 -> [w353 _]
                  tunnel: w337 -> [w352 _]
                  frame No Error {
                    n158 = Unbundle(w356) -> ("Calibration Quality"=w357:dbl)  [unwired: 3 out]
                    n159 = Greater Or Equal?(x=w357, y=0.2) -> (x >= y?=w354:bool)
                    n160 = case shown="True" w354 {
                      tunnel: [w359 w366] -> w355
                      tunnel: w353 -> [_ w365]
                      tunnel: w352 -> [_ w361]
                      frame False {
                        w359 = u16 1  # Calibrating
                      }
                      frame True {
                        w366 = u16 2  # System Calibrated
                        n161 = call "IMAQ Get Binocular Stereo Calibration Info"("Binocular Stereo Session"=w365) -> ("Q Matrix"=w364:dbl[][], "error out"=w363:errorcluster)  [unwired: 1 in, 12 out]
                        n162 = call "IMAQ Get Maximum Disparity 2"("error in (no error)"=w363, "Image Width (pixels)"=w361, "Min. Desired Depth (units)"=15.0, "Q Matrix"=w364) -> ("Max. Disparity"=w362:i32)  [unwired: 5 in, 2 out]
                        n163 = property on="Number of Disparity" class="DigNum (strict)"("Value"=w362) -> ()  [unwired: 2 in, 2 out]
                        n164 = property on="Number of Disparity" class="DigNum (strict)"("Value"=w362) -> ()  [unwired: 2 in, 2 out]
                      }
                    }
                  }
                  frame Error {
                    w367 = u16 0  # System not Calibrated
                    n165 = call <vilib>:"General Error Handler.vi"("error in (no error)"=w368) -> ()  [unwired: 2 in, 13 out]
                  }
                }
                n166 = local write "Calibration Status"(w346) -> ()
              }
              frame #3 {
                n167 = case shown="2" w370 {
                  frame 0, Default {
                  }
                  frame 2 {
                    w371 = T15."Enabled" ("Disabled")
                    w374 = T16."Page Enabled" ("Page Enabled State")
                    n168 = property on="Tab" class="TabCtl (strict)"() -> ("Pages"=w378:refnum<vi>[])  [unwired: 2 in, 2 out]
                    n169 = Index Array(array=w378, index #1=1 ("index"), index #2=2 ("index")) -> (element #1=w377:refnum<vi>, element #2=w373:refnum<vi>)
                    n170 = property on="Scaling Factor" class="DigNum (strict)"("Disabled"=w371) -> ()  [unwired: 2 in, 2 out]
                    n171 = property on="Save Stereo Calibration" class="Bool"("Disabled"=w371) -> ()  [unwired: 2 in, 2 out]
                    n172 = property on="View" class="Enum (strict)"("Disabled"=w371, "Val(Sgnl)"=enum16{"Acquired Images", "Rectified Images"}."Rectified Images" ("View")) -> ()  [unwired: 2 in, 2 out]
                    n173 = property class="Page"(reference=w377, "PageEnb"=w374) -> ()  [unwired: 1 in, 2 out]
                    n174 = property class="Page"(reference=w373, "PageEnb"=w374) -> ()  [unwired: 1 in, 2 out]
                  }
                }
                n175 = property on="Calibration Status" class="Ring (strict)"("Blinking"=FALSE) -> ()  [unwired: 2 in, 2 out]
              }
            }
          }
          event "Load": Value Change {
            n176 = event-data() -> ()  [unwired: 2 out]
            n177 = call "File Dialog2"("prompt"="Select a stereo calibration file") -> ("selected path"=w382:path, "cancelled"=w381:bool, "error out"=w379:errorcluster)  [unwired: 6 in, 6 out]
            n178 = case shown="False" w381 {
              tunnel: w383 -> [w386 _]
              tunnel: w382 -> [w384 _]
              tunnel: w379 -> [_ _]
              frame False {
                n179 = call "IMAQ Read Binocular Stereo File"("File Path"=w384, "Binocular Stereo Session (optional)"=w386) -> ("error out"=w385:errorcluster)  [unwired: 1 in, 8 out]
                n180 = case shown="No Error" w385 {
                  selector: w385 -> [_ w396]
                  frame No Error {
                    w390 = T16."Page Enabled" ("Page Enabled State")
                    w395 = u16 2  # System Calibrated
                    n181 = property on="Tab" class="TabCtl (strict)"() -> ("Pages"=w394:refnum<vi>[])  [unwired: 2 in, 2 out]
                    n182 = property on="View" class="Enum (strict)"() -> ("Value"=w388:enum16{"Acquired Images", "Rectified Images"})  [unwired: 2 in, 2 out]
                    n183 = Index Array(array=w394, index #1=1 ("index"), index #2=2 ("index")) -> (element #1=w393:refnum<vi>, element #2=w389:refnum<vi>)  [unwired: 1 in, 1 out]
                    n184 = local write "Calibration Status"(w395) -> ()
                    n185 = property on="View" class="Enum (strict)"("Disabled"=T15."Enabled", "Val(Sgnl)"=w388) -> ()  [unwired: 2 in, 2 out]
                    n186 = property class="Page"(reference=w393, "PageEnb"=w390) -> ()  [unwired: 1 in, 2 out]
                    n187 = property class="Page"(reference=w389, "PageEnb"=w390) -> ()  [unwired: 1 in, 2 out]
                  }
                  frame Error {
                    n188 = call <vilib>:"General Error Handler.vi"("error in (no error)"=w396) -> ()  [unwired: 2 in, 13 out]
                  }
                }
              }
              frame True {
              }
            }
          }
          event "Save Stereo Calibration": Value Change {
            n189 = event-data() -> ()  [unwired: 2 out]
            n190 = call "File Dialog"("prompt"="Save Stereo Calibration File As...") -> ("selected path"=w399:path, "cancelled"=w398:bool)  [unwired: 6 in, 7 out]
            n191 = case shown="False" w398 {
              tunnel: w397 -> [w402 _]
              tunnel: w399 -> [w401 _]
              frame False {
                n192 = call "IMAQ Write Binocular Stereo File"("File Path"=w401, "Binocular Stereo Session"=w402) -> ()  [unwired: 3 in, 7 out]
              }
              frame True {
              }
            }
          }
          event "Save Grid Images": Value Change {
            n193 = event-data() -> ()  [unwired: 2 out]
            n194 = call "File Dialog3"("prompt"="Save Grid Images in...") -> ("selected path"=w404:path, "cancelled"=w403:bool)  [unwired: 6 in, 7 out]
            n195 = case shown="False" w403 {
              tunnel: w404 -> [w406 _]
              frame False {
                n196 = call "Stereo - Calibration Manager.vi"("Function"=Stereo_-_Calibration_Manager_Function."Get Images") -> ("Grid Images out"=w407:cluster{"Left Image":T4, "Right Image":T4}[])  [unwired: 2 in, 8 out]
                n197 = for {
                  tunnel: w407 -> [w419] mode=indexing
                  tunnel: w406 -> [w414]
                  i -> [w410]
                  n198 = Format Into String(format string="Left Grid %d.png", w410) -> (resulting string=w415:string)  [unwired: 2 in, 1 out]
                  n199 = Format Into String(format string="Right Grid %d.png", w410) -> (resulting string=w412:string)  [unwired: 2 in, 1 out]
                  n200 = Build Path(base path=w414, name or relative path=w415) -> (appended path=w411:path)
                  n201 = Build Path(base path=w414, name or relative path=w412) -> (appended path=w409:path)
                  n202 = Unbundle By Name(w419) -> ("Left Image"=w418:T4, "Right Image"=w417:T4)
                  n203 = call-poly "IMAQ Write File 2"("File Path"=w411, "Image"=w418) -> ()  [unwired: 4 in, 6 out]
                  n204 = call-poly "IMAQ Write File 2"("File Path"=w409, "Image"=w417) -> ()  [unwired: 4 in, 6 out]
                }
              }
              frame True {
              }
            }
          }
          event "Save Single Calibrations": Value Change {
            n205 = event-data() -> ()  [unwired: 2 out]
            n206 = call "File Dialog4"("prompt"="Save Single Calibration Templates in...") -> ("selected path"=w421:path, "cancelled"=w420:bool)  [unwired: 6 in, 7 out]
            n207 = case shown="False" w420 {
              tunnel: w421 -> [w425 _]
              frame False {
                n208 = call "Stereo - Calibration Manager.vi"("Function"=Stereo_-_Calibration_Manager_Function."Get Images") -> ("Calibrated Images"=w424:T4[])  [unwired: 2 in, 8 out]
                n209 = for {
                  tunnel: w425 -> [w430]
                  tunnel: w424 -> [w429] mode=indexing
                  tunnel: string[] ["Left Single Calibration Template.png", "Right Single Calibration Template.png"] -> [w427] mode=indexing
                  n210 = Build Path(base path=w430, name or relative path=w427) -> (appended path=w428:path)
                  n211 = call-poly "IMAQ Write File 2"("File Path"=w428, "Image"=w429) -> ()  [unwired: 2 in, 8 out]
                }
              }
              frame True {
              }
            }
          }
          event "View": Value Change {
            n212 = event-data() -> ("NewVal"=w432:enum16{"Acquired Images", "Rectified Images"})  [unwired: 1 out]
            n213 = Equal?(x=w432, y=enum16{"Acquired Images", "Rectified Images"}."Rectified Images" ("View")) -> (x = y?=w436:bool)
            n214 = Select(t=u8 0 ("Disabled"), s=w436, f=u8 2) -> (s? t:f=w435:u8)
            n215 = property on="Overlay Horizontal Lines" class="Bool (strict)"("Disabled"=w435) -> ()  [unwired: 2 in, 2 out]
          }
          event "Filter Cap", "Postfilter Options SGBM", "Correspondence Options SGBM", "Prefilter Options", "Postfilter Options BM", "Correspondence Options BM", "Interpolate Disparity", "Process Band": Value Change {
            n216 = event-data() -> ()  [unwired: 2 out]
            n217 = local read "Tab Control"() -> (w449:T3)
            n218 = case shown="\"Semi Global Block Matching Algorithm\", \"Block Matching Algorithm\"" w449 {
              selector: w449 -> [_ w486]
              tunnel: w461 -> [_ w467]
              tunnel: w460 -> [_ w495]
              tunnel: w459 -> [_ w494]
              tunnel: w458 -> [_ w493]
              tunnel: "Postfilter Options BM" -> [_ w492]
              tunnel: "Prefilter Options" -> [_ w491]
              tunnel: "Correspondence Options BM" -> [_ w490]
              tunnel: "Postfilter Options SGBM" -> [_ w489]
              tunnel: "Filter Cap" -> [_ w488]
              tunnel: "Correspondence Options SGBM" -> [_ w487]
              tunnel: [w462 w480] -> w439
              tunnel: w451 -> [_ w471]
              tunnel: [FALSE ("Visible") TRUE ("Visible")] -> w450
              tunnel: [FALSE ("Visible") TRUE ("Visible")] -> w437
              tunnel: ["Grid Coverage" ("Caption.Text") w470] -> w448
              tunnel: [w463 u8 0 ("Disabled")] -> w447
              tunnel: "Interpolate Disparity" -> [_ w468]
              tunnel: "Process Band" -> [_ w479]
              frame "Stereo System Calibration", Default {
                n219 = property on="View" class="Enum (strict)"() -> ("Disabled"=w463:u8)  [unwired: 2 in, 2 out]
                n220 = property on="Image" class="IntGraph (strict)"() -> ("Value"=w462:sgl[][])  [unwired: 2 in, 2 out]
              }
              frame "Semi Global Block Matching Algorithm", "Block Matching Algorithm" {
                n221 = case shown="\"Semi Global Block Matching Algorithm\"" w486 {
                  tunnel: w467 -> [w536 w549]
                  tunnel: w495 -> [w535 w547]
                  tunnel: w494 -> [w534 w546]
                  tunnel: w493 -> [w533 w548]
                  tunnel: [w532 w545] -> w478
                  tunnel: w492 -> [w531 _]
                  tunnel: w491 -> [w530 _]
                  tunnel: w490 -> [w528 _]
                  tunnel: w489 -> [_ w544]
                  tunnel: w488 -> [_ w543]
                  tunnel: w487 -> [_ w541]
                  tunnel: [w529 w542] -> w476
                  tunnel: [w527 w540] -> w472
                  tunnel: [w526 w539] -> w477
                  tunnel: [w525 w538] -> w481
                  tunnel: w479 -> [w524 w537]
                  frame "Block Matching Algorithm", Default {
                    n222 = call "IMAQ Stereo Correspondence (Block Matching)"("Binocular Stereo Session"=w536, "Prefilter Options"=w530, "Postfilter Options"=w531, "Process Band?"=w524, "Left Image In"=w535, "Right Image In"=w534, "Disparity Image In"=w533, "Correspondence Options"=w528) -> ("Disparity Image Out"=w532:T4, "error out"=w529:errorcluster)  [unwired: 2 in, 4 out]
                    n223 = Unbundle(w528) -> ("Minimum Disparity"=w526:dbl, "Number of Disparity"=w525:dbl, "Invalid Disparity Replace Value"=w527:dbl)  [unwired: 4 out]
                  }
                  frame "Semi Global Block Matching Algorithm" {
                    n224 = call "IMAQ Stereo Correspondence (SG Block Matching)"("Binocular Stereo Session"=w549, "Filter Cap"=w543, "Postfilter Options"=w544, "Process Band?"=w537, "Left Image In"=w547, "Right Image In"=w546, "Disparity Image In"=w548, "Correspondence Options"=w541) -> ("Disparity Image Out"=w545:T4, "error out"=w542:errorcluster)  [unwired: 2 in, 4 out]
                    n225 = Unbundle(w541) -> ("Minimum Disparity"=w539:dbl, "Number of Disparity"=w538:dbl, "Invalid Disparity Replace Value"=w540:dbl)  [unwired: 7 out]
                  }
                }
                n226 = case shown="True" w468 {
                  tunnel: w478 -> [w514 w523]
                  tunnel: [w514 w522] -> w475
                  tunnel: w472 -> [_ w521]
                  tunnel: w477 -> [_ w520]
                  tunnel: w481 -> [_ w519]
                  tunnel: w476 -> [w513 w516]
                  tunnel: [w513 w515] -> w473
                  frame False {
                  }
                  frame True {
                    n227 = call "IMAQ Interpolate Disparity Image"("Sampling Frequency"=25, "Number of Disparities"=w519, "Order"=12, "Minimum Disparity"=w520, "error in (no error)"=w516, "Invalid Disparity Value"=w521, "Image Src"=w523) -> ("error out"=w515:errorcluster, "Image Dst Out"=w522:T4)  [unwired: 1 in, 2 out]
                  }
                }
                n228 = case shown="\"Disparity Image\", Default" "Display" {
                  tunnel: [w501 w506] -> w482
                  tunnel: w475 -> [w503 w512]
                  tunnel: w467 -> [_ w511]
                  tunnel: w473 -> [w502 w510]
                  tunnel: w472 -> [_ w509]
                  tunnel: w471 -> [_ w508]
                  tunnel: ["Disparity Image" ("Caption.Text") "Depth Image" ("Caption.Text")] -> w470
                  frame "Disparity Image", Default {
                    n229 = call "IMAQ ImageToArray"("error in (no error)"=w502, "Image"=w503) -> ("Image Pixels (I16)"=w501:i16[][])  [unwired: 1 in, 5 out]
                  }
                  frame "Depth Image" {
                    n230 = call "IMAQ Get Depth Image From Stereo"("Invalid Disparity Value"=w509, "error in (no error)"=w510, "Depth Image In"=w508, "Disparity Image"=w512, "Binocular Stereo Session"=w511) -> ("error out"=w505:errorcluster, "Depth Image Out"=w507:T4)  [unwired: 2 in, 3 out]
                    n231 = call "IMAQ ImageToArray"("error in (no error)"=w505, "Image"=w507) -> ("Image Pixels (Float)"=w506:sgl[][])  [unwired: 1 in, 5 out]
                  }
                }
                n232 = local read "Process Band"() -> (w469:bool)
                n233 = case shown="False" w469 {
                  tunnel: w482 -> [w498 w499]
                  tunnel: w481 -> [w497 _]
                  tunnel: [w496 w499] -> w480
                  frame False {
                    n234 = Array Subset(array=w498, index (col)=w497) -> (w496:sgl[][])  [unwired: 3 in]
                  }
                  frame True {
                  }
                }
              }
            }
            "Image" <- w439
            n235 = property on="View" class="Enum (strict)"("Disabled"=w447) -> ("Value"=w446:enum16{"Acquired Images", "Rectified Images"})  [unwired: 2 in, 2 out]
            n236 = property on="Image" class="IntGraph (strict)"("Visible"=w450, "Caption.Text"=w448) -> ()  [unwired: 2 in, 2 out]
            n237 = property on="Live Image" class="Bool (strict)"("Visible"=w437) -> ()  [unwired: 2 in, 2 out]
            n238 = property on="Display" class="Enum (strict)"("Visible"=w437) -> ()  [unwired: 2 in, 2 out]
            n239 = property on="Relative Coordinate System" class="Clust (strict)"("Visible"=w437) -> ()  [unwired: 2 in, 2 out]
            n240 = property on="Interpolate Disparity" class="Bool (strict)"("Visible"=w437) -> ()  [unwired: 2 in, 2 out]
            n241 = property on="Process Band" class="Bool (strict)"("Visible"=w437) -> ()  [unwired: 2 in, 2 out]
            n242 = property on="Depth" class="DigNum (strict)"("Visible"=w437) -> ()  [unwired: 2 in, 2 out]
            n243 = property on="Unit" class="Str"("Visible"=w437) -> ()  [unwired: 2 in, 2 out]
            n244 = Equal?(x=enum16{"Acquired Images", "Rectified Images"}."Rectified Images" ("View"), y=w446) -> (x = y?=w444:bool)
            n245 = Select(t=u8 0 ("Disabled"), s=w444, f=u8 2) -> (s? t:f=w443:u8)
            n246 = property on="Overlay Horizontal Lines" class="Bool (strict)"("Disabled"=w443) -> ()  [unwired: 2 in, 2 out]
          }
          event "Tab Control", "Correspondence Options SGBM.Minimum Disparity", "Correspondence Options SGBM.Number of Disparity", "Correspondence Options BM.Minimum Disparity", "Correspondence Options BM.Number of Disparity", "Display", "Max Depth (SGBM)", "Max Depth (BM)": Value Change {
            n247 = event-data() -> ()  [unwired: 2 out]
            n248 = local read "Tab Control"() -> (w553:T3)
            n249 = local read "Display"() -> (w551:enum16{"Disparity Image", "Depth Image"})
            n250 = local read "Interpolate Disparity"() -> (w550:bool)
            n251 = case shown="\"Disparity Image\", Default" w551 {
              tunnel: [w559 w572] -> w556
              tunnel: w553 -> [w560 w578]
              tunnel: [w558 w574] -> w555
              tunnel: u32[] [0, 7, 15, 22, 29, 36, 44, 51, 58, 66, 73, 80, 87, 95, 102, 109, 117, 124, 131, 138, 146, 153, 160, 168, 175, 182, 189, 197, 204, 211, 219, 226, 233, 240, 248, 255, 75263, 76799, 78335, 79871, 81407, 82943, 84479, 86015, 87551, 89087, 90623, 92159, 93695, 95231, 96767, 98303, 99839, 101375, 102911, 104447, 105983, 107519, 109055, 110591, 112127, 113663, 115199, 116735, 118271, 119807, 121343, 122879, 124415, 125951, 127487, 129023, 130559, 131069, 131063, 131057, 131051, 131045, 131039, 131033, 131027, 131021, 131015, 131009, 131003, 130997, 130991, 130985, 130979, 130973, 130967, 130961, 130955, 130949, 130943, 130937, 130931, 130925, 130919, 130913, 130907, 130901, 130895, 130889, 130883, 130877, 130871, 130865, 130859, 130853, 130847, 130841, 130835, 130829, 130823, 130817, 524033, 917249, 1310465, 1703681, 2096897, 2490113, 2883329, 3276545, 3669761, 4062977, 4456193, 4849409, 5242625, 5635841, 6029057, 6422273, 6815489, 7208705, 7601921, 7995137, 8388353, 8781569, 9174785, 9568001, 9961217, 10354433, 10747649, 11140865, 11534081, 11927297, 12320513, 12713729, 13106945, 13500161, 13893377, 14286593, 14679809, 15073025, 15466241, 15859457, 16252673, 16645889, 16776449, 16774913, 16773377, 16771841, 16770305, 16768769, 16767233, 16765697, 16762625, 16761089, 16759553, 16758017, 16756481, 16754945, 16753409, 16751873, 16750337, 16748801, 16747265, 16745729, 16744193, 16742657, 16741121, 16739585, 16738049, 16736513, 16734977, 16733441, 16731905, 16730369, 16728833, 16727297, 16725761, 16724225, 16722689, 16721153, 16719617, 16718081, 16716545, 16715009, 16713473, 16711937, 16711937, 16711943, 16711949, 16711955, 16711961, 16711967, 16711973, 16711979, 16711985, 16711991, 16711997, 16712003, 16712009, 16712015, 16712021, 16712027, 16712033, 16712039, 16712045, 16712051, 16712057, 16712063, 16712069, 16712075, 16712081, 16712087, 16712093, 16712099, 16712105, 16712111, 16712117, 16712123, 16712129, 16712135, 16712141, 16712147, 16712153, 16712159, 16712165, 16712171, 16712177, 16712183, 16712189, 16581119, 16187903, 15794687, 15401471, 15008255, 14615039, 14221823, 13828607, 13435391, 13042175, 12648959, 12255743, 11862527] ("appended array") -> [w557 w571]
              tunnel: [w557 w570] -> w554
              frame "Disparity Image", Default {
                w561 = 16.0 ("y")
                n252 = case shown="\"Block Matching Algorithm\"" w560 {
                  tunnel: [w565 w568] -> w563
                  tunnel: [w564 w567] -> w562
                  frame "Semi Global Block Matching Algorithm", Default {
                    n253 = local read "Correspondence Options SGBM"() -> (w566:T7)
                    n254 = Unbundle By Name(w566) -> ("Minimum Disparity"=w565:dbl, "Number of Disparity"=w564:dbl)
                  }
                  frame "Block Matching Algorithm" {
                    n255 = local read "Correspondence Options BM"() -> (w569:T9)
                    n256 = Unbundle By Name(w569) -> ("Minimum Disparity"=w568:dbl, "Number of Disparity"=w567:dbl)
                  }
                }
                n257 = Multiply(x=w561, y=w563) -> (x*y=w559:dbl)
                n258 = Multiply(x=w562, y=w561) -> (x*y=w558:dbl)
              }
              frame "Depth Image" {
                n259 = case shown="\"Semi Global Block Matching Algorithm\", Default" w578 {
                  tunnel: ["Max Depth (SGBM)" "Max Depth (BM)"] -> w574
                  frame "Semi Global Block Matching Algorithm", Default {
                  }
                  frame "Block Matching Algorithm" {
                  }
                }
                n260 = Reverse 1D Array(array=w571) -> (reversed array=w570:u32[])
                n261 = Multiply(x=w574, y=sgl 20.0) -> (x*y=w576:sgl)
                n262 = Divide(x=w576, y=sgl 100.0) -> (x/y=w573:sgl)
                n263 = Subtract(x=w574, y=w573) -> (x-y=w572:sgl)
              }
            }
            n264 = property on="Interpolate Disparity" class="Bool (strict)"("Val(Sgnl)"=w550) -> ()  [unwired: 2 in, 2 out]
            n265 = property on="Image" class="IntGraph (strict)"("ZScale.Minimum"=w556, "ZScale.Maximum"=w555) -> ()  [unwired: 2 in, 2 out]
            n266 = property on="Image" class="IntGraph (strict)"("Color Table"=w554) -> ()  [unwired: 2 in, 2 out]
          }
          event "Image": Mouse Move {
            n267 = event-data() -> ("CtlRef"=w590:refnum<vi>, "Coords"=w589:T22)  [unwired: 1 out]
            n268 = local read "Tab Control"() -> (w594:T3)
            n269 = case shown="\"Semi Global Block Matching Algorithm\", Default" w594 {
              tunnel: [w601 w605] -> w592
              tunnel: [w599 w603] -> w586
              tunnel: [w598 w602] -> w581
              frame "Semi Global Block Matching Algorithm", Default {
                n270 = local read "Correspondence Options SGBM"() -> (w600:T7)
                n271 = Unbundle By Name(w600) -> ("Invalid Disparity Replace Value"=w598:dbl, "Number of Disparity"=w599:dbl)
                n272 = local read "Max Depth (SGBM)"() -> (w601:sgl)
              }
              frame "Block Matching Algorithm" {
                n273 = local read "Correspondence Options BM"() -> (w604:T9)
                n274 = Unbundle By Name(w604) -> ("Invalid Disparity Replace Value"=w602:dbl, "Number of Disparity"=w603:dbl)
                n275 = local read "Max Depth (BM)"() -> (w605:sgl)
              }
            }
            n276 = invoke class="IntGraph (strict)" method="Map Coords To XY"(reference=w590, "Coords"=w589) -> ("XY"=w588:cluster{"X":dbl, "Y":dbl})  [unwired: 5 in, 6 out]
            n277 = Bundle By Name(cluster=cluster{"X":dbl, "Y":dbl} {"X"=0.0, "Y"=0.0} ("y"), "X"=w586) -> (w584:cluster{"X":dbl, "Y":dbl})
            n278 = Bundle("Max Depth (BM)"=sgl 0.0, "Max Depth (BM)"=w592) -> (w591:T23)  [unwired: 1 out]
            n279 = Add(x=w588, y=w584) -> (x+y=w587:cluster{"X":dbl, "Y":dbl})
            n280 = call "IMAQ Convert Pixel To 3D Coordinates"("Binocular Stereo Session"=w597, "Relative Coordinate System"="Relative Coordinate System", "Invalid Disparity Value"=w581, "Disparity Image"=w596, "Pixel Coordinates"=w587, "Depth Control"=w591) -> ("Real World 3D Coordinates"=w583:cluster{"X":dbl, "Y":dbl, "Z":dbl})  [unwired: 2 in, 7 out]
            n281 = Unbundle By Name(w583) -> ("Z"=→"Depth":dbl)
          }
        }
      }
    }
    frame #3 {
      # "Dispose of the session and images"
      n282 = Build Array(w612, w611, w610, w609, w608, w606) -> (w607:T4[])
      n283 = for {
        tunnel: w607 -> [w614] mode=indexing
        n284 = call "IMAQ Dispose"("Image"=w614) -> ()  [unwired: 2 in, 4 out]
      }
      n285 = call "IMAQ Dispose Binocular Stereo Session"("Binocular Stereo Session"=w613) -> ()  [unwired: 1 in, 10 out]
    }
  }
